vi "Update.vi"(8 "error in (no error)":errorcluster, 10 "Message in":refnum<class "UpdateMessage.lvclass">, 11 "RSA in":refnum<class "RSA.lvclass">) -> (0 "error out":errorcluster, 3 "RSA out":refnum<class "RSA.lvclass">)   [LabVIEW 2012, in "RSA.lvclass"]
doc: "The update method processes the command 'update'. \n\nThe command 'update' is used for receiving new values to be set to the private data of the class. This could be seen as a public set method for setting new parameters to the private class data."
uses:
  RSA.lvclass
  <vilib>/Distrio/Murmex/UpdateMessage/UpdateMessage.lvclass
  RSA.lvclass/RSA.ctl
  starting shape.ctl
  <vilib>/Distrio/Murmex/Murmex/Murmex.lvclass
panel:
  # "This method is called when the UPDATE\ntrigger is sent. \n\nOverride this method when your component needs to\nrespond to this trigger. \n\nCall parent for proper implementation"
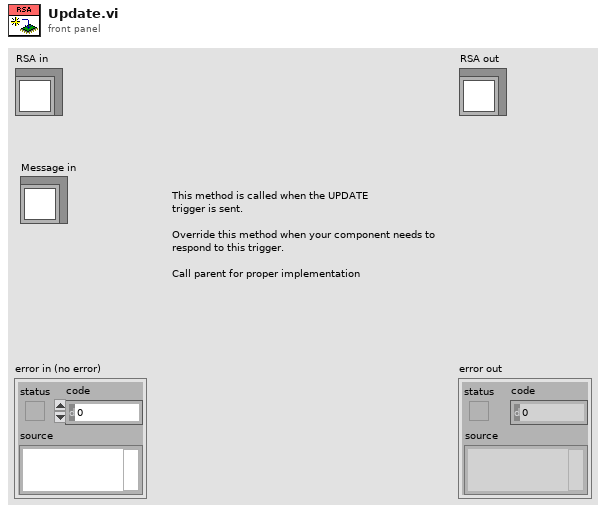
[diagram p1: front panel]
types:
  T1 = typedef "RSA.lvclass/starting shape.ctl" = enum16{"Load shape", "Midrange"}
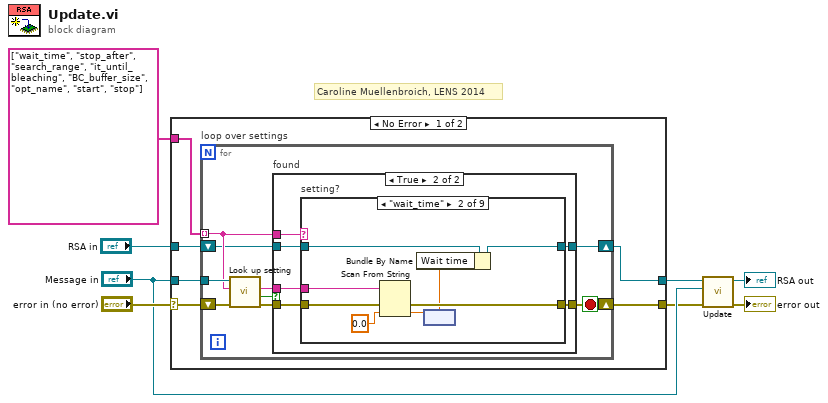
[diagram p0: block diagram]
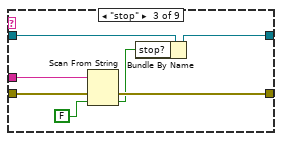
[diagram p4: hidden frame]
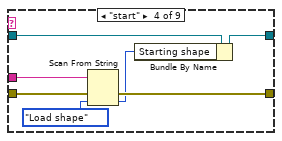
[diagram p5: hidden frame]
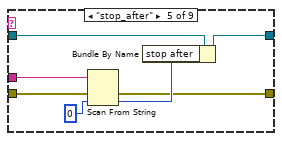
[diagram p6: hidden frame]
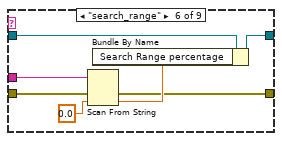
[diagram p7: hidden frame]
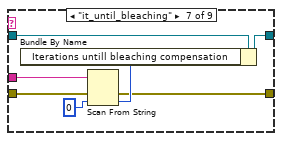
[diagram p8: hidden frame]
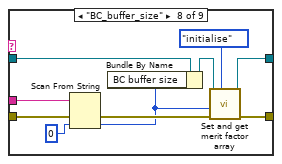
[diagram p9: hidden frame]
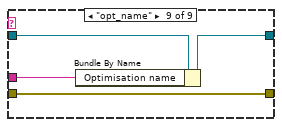
[diagram p10: hidden frame]
diagram:
  # "Caroline Muellenbroich, LENS 2014"
  n1 = case shown="No Error" "error in (no error)" {
    selector: "error in (no error)" -> [w14 w92]
    tunnel: "Message in" -> [w13 _]
    tunnel: string[] ["wait_time", "stop_after", "search_range", "it_until_bleaching", "BC_buffer_size", "opt_name", "start", "stop"] ("key chains") -> [w12 _]
    tunnel: "RSA in" -> [w11 w91]
    tunnel: [w10 w92] -> w3
    tunnel: [w9 w91] -> w2
    frame No Error {
      n2 = for "loop over settings" {
        shift-right: [w15] -> w10
        shift-left: w14 -> [w23]
        tunnel: w13 -> [w22]
        tunnel: w12 -> [w19] mode=indexing
        shift-right: [w18] -> w9
        shift-left: w11 -> [w17]
        stop <- w15 stop-if-true
        n3 = call <vilib>:"Look up setting.vi"("error in (no error)"=w23, "tag name"=w19, "UpdateMessage in"=w22) -> ("error out"=w16:errorcluster, "found?"=w21:bool, "value"=w20:string)  [unwired: 5 in, 1 out]
        n4 = case "found" shown="True" w21 {
          tunnel: w20 -> [_ w30]
          tunnel: w19 -> [_ w31]
          tunnel: [w24 w29] -> w18
          tunnel: w17 -> [w24 w28]
          tunnel: w16 -> [w25 w27]
          tunnel: [w25 w26] -> w15
          frame False {
          }
          frame True {
            n5 = case "setting?" shown="\"wait_time\"" w31 {
              tunnel: w30 -> [_ w41 w48 w55 w62 w69 w76 w86 w89]
              tunnel: [w33 w40 w47 w54 w61 w68 w75 w81 w90] -> w29
              tunnel: w28 -> [w33 w39 w46 w53 w60 w63 w74 w85 w87]
              tunnel: [w32 w36 w44 w51 w56 w64 w70 w79 w88] -> w26
              tunnel: w27 -> [w32 w37 w45 w52 w57 w65 w71 w83 w88]
              frame "False", Default {
              }
              frame "wait_time" {
                n6 = Scan From String(input string=w41, error in=w37, default 1=0.0 ("Settings Cluster.Wait time")) -> (error out=w36:errorcluster, output 1=w35:dbl)  [unwired: 2 in, 2 out]
                n7 = node(w35) -> (w34:dbl[unit])
                n8 = Bundle By Name(cluster=w39, "Wait time"=w34) -> (w40:refnum<class "RSA.lvclass">)
              }
              frame "stop" {
                n9 = Scan From String(input string=w48, error in=w45, default 1=FALSE ("Run time cluster.stop?")) -> (error out=w44:errorcluster, output 1=w42:bool)  [unwired: 2 in, 2 out]
                n10 = Bundle By Name(cluster=w46, "stop?"=w42) -> (w47:refnum<class "RSA.lvclass">)
              }
              frame "start" {
                n11 = Scan From String(input string=w55, error in=w52, default 1=starting_shape."Load shape" ("Settings Cluster.Starting shape")) -> (error out=w51:errorcluster, output 1=w49:T1)  [unwired: 2 in, 2 out]
                n12 = Bundle By Name(cluster=w53, "Starting shape"=w49) -> (w54:refnum<class "RSA.lvclass">)
              }
              frame "stop_after" {
                n13 = Scan From String(input string=w62, error in=w57, default 1=0 ("Settings Cluster.stop after")) -> (error out=w56:errorcluster, output 1=w59:i32)  [unwired: 2 in, 2 out]
                n14 = Bundle By Name(cluster=w60, "stop after"=w59) -> (w61:refnum<class "RSA.lvclass">)
              }
              frame "search_range" {
                n15 = Scan From String(input string=w69, error in=w65, default 1=0.0 ("Settings Cluster.stop after")) -> (error out=w64:errorcluster, output 1=w67:dbl)  [unwired: 2 in, 2 out]
                n16 = Bundle By Name(cluster=w63, "Search Range percentage"=w67) -> (w68:refnum<class "RSA.lvclass">)
              }
              frame "it_until_bleaching" {
                n17 = Scan From String(input string=w76, error in=w71, default 1=0 ("Settings Cluster.stop after")) -> (error out=w70:errorcluster, output 1=w73:i32)  [unwired: 2 in, 2 out]
                n18 = Bundle By Name(cluster=w74, "Iterations untill bleaching compensation"=w73) -> (w75:refnum<class "RSA.lvclass">)
              }
              frame "BC_buffer_size" {
                n19 = Scan From String(input string=w86, error in=w83, default 1=0 ("Settings Cluster.stop after")) -> (error out=w80:errorcluster, output 1=w77:i32)  [unwired: 2 in, 2 out]
                n20 = Bundle By Name(cluster=w85, "BC buffer size"=w77) -> (w82:refnum<class "RSA.lvclass">)
                n21 = call "Set and get merit factor array.vi"("action"=enum16{"set", "get", "initialise"}."initialise", "error in (no error)"=w80, "array size"=w77, "RSA in"=w82) -> ("error out"=w79:errorcluster, "RSA out"=w81:refnum<class "RSA.lvclass">)  [unwired: 4 in, 2 out]
              }
              frame "opt_name" {
                n22 = Bundle By Name(cluster=w87, "Optimisation name"=w89) -> (w90:refnum<class "RSA.lvclass">)
              }
            }
          }
        }
      }
    }
    frame Error {
    }
  }
  n23 = call-parent "Update.vi"("error in (no error)"=w3, "Message in"="Message in", "Murmex in"=w2) -> ("error out"=→"error out":errorcluster, "Murmex out"=→"RSA out":refnum<class "RSA.lvclass">)  [unwired: 7 in]
